vi "Write AllClasses.vi"(8 "error in (no error)":errorcluster, 10 "AllClasses":refnum<class "baseClass.lvclass">[](array[class]), 11 "baseParser in":refnum<class "baseParser.lvclass">) -> (0 "error out":errorcluster, 3 "baseParser out":refnum<class "baseParser.lvclass">)   [LabVIEW 2013, in "baseParser.lvclass"]
uses:
  baseParser.lvclass
  baseClass/baseClass.lvclass
  baseParser.lvclass/baseParser.ctl
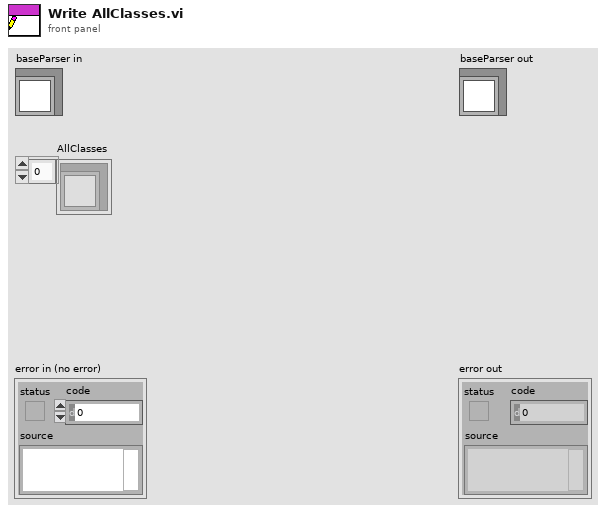
[diagram p1: front panel]
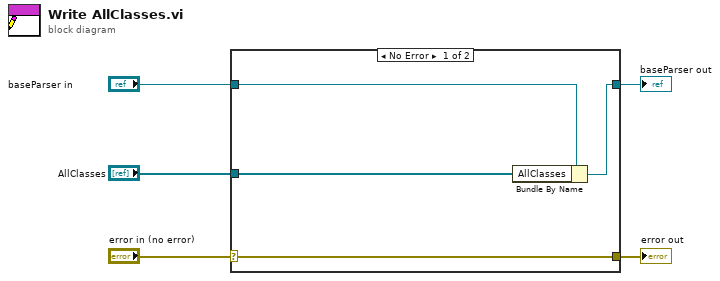
[diagram p0: block diagram]
diagram:
  n1 = case shown="No Error" "error in (no error)" {
    selector: "error in (no error)" -> [w9 w10]
    tunnel: [w9 w10] -> w4
    tunnel: [w7 w11] -> w2
    tunnel: "baseParser in" -> [w8 w11]
    tunnel: "AllClasses" -> [w6 _]
    frame No Error {
      n2 = Bundle By Name(cluster=w8, "AllClasses"=w6) -> (w7:refnum<class "baseParser.lvclass">)
    }
    frame Error {
    }
  }
  "error out" <- w4
  "baseParser out" <- w2
